vi "Get Interface Info.vi"(8 "error in (no error)":errorcluster, 10 "CASE":string, 11 "CSM-Helper in":refnum<class "CSM-Helper.lvclass">) -> (0 "error out":errorcluster, 1 "Response":T1[](array[typedef]), 2 "Array":T1[](array[typedef]), 3 "CSM-Helper out":refnum<class "CSM-Helper.lvclass">)   [LabVIEW 2017, in "CSM-Helper.lvclass"]
uses:
  CSM-Helper.lvclass
  Typedef/Def-Argument Info.ctl
  CSM-Helper.lvclass/CSM-Helper.ctl
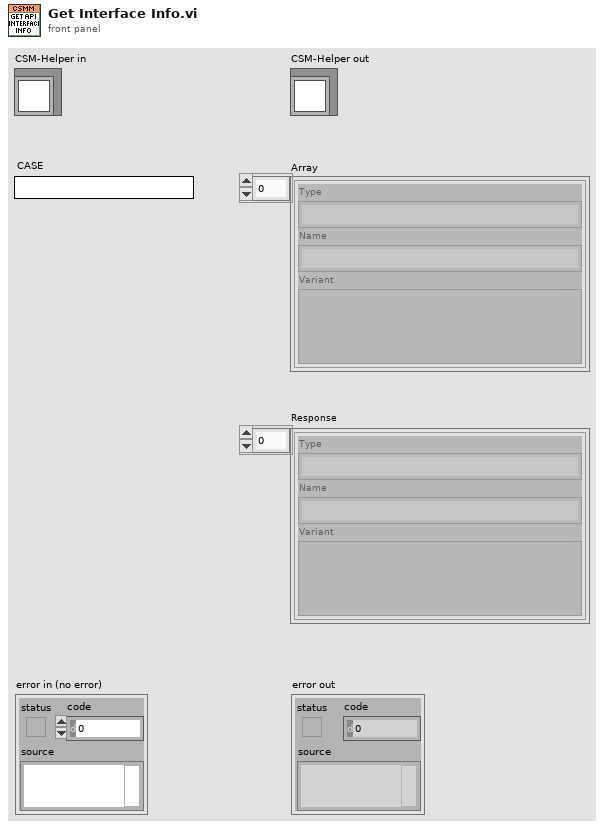
[diagram p1: front panel]
types:
  T1 = typedef "CSM-Helper.lvclass/Def-Argument Info.ctl" = cluster{"Type":string, "Name":string, "Variant":variant}
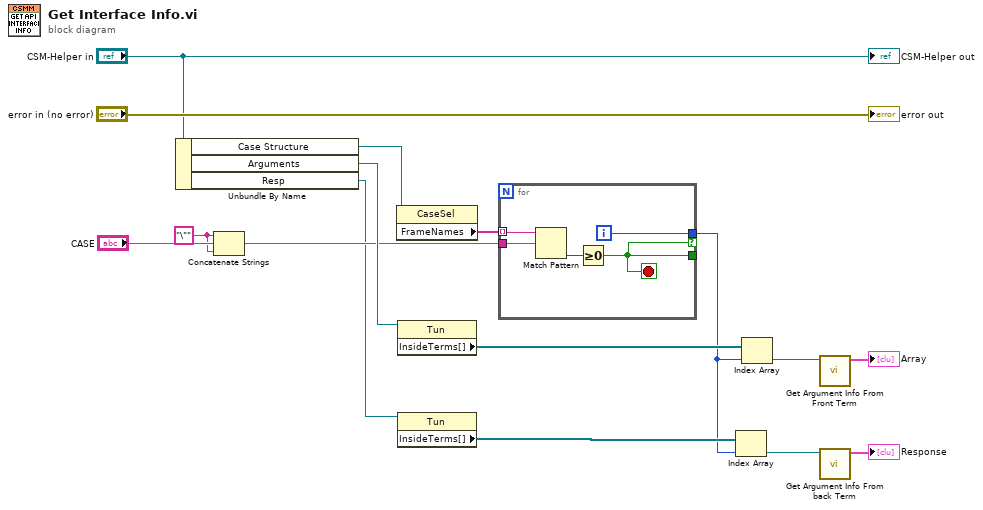
[diagram p0: block diagram]
diagram:
  w9 = "\"" ("string")
  n1 = Unbundle By Name("CSM-Helper in") -> ("Case Structure"=w14:refnum<vi>, "Arguments"=w13:refnum<vi>, "Resp"=w6:refnum<vi>)
  n2 = Concatenate Strings(w9, "CASE", w9) -> (w10:string)
  n3 = property class="CaseSel"(reference=w14) -> ("FrameNames"=w12:string[])  [unwired: 1 in, 2 out]
  n4 = property class="Tun"(reference=w13) -> ("InsideTerms[]"=w8:refnum<vi>[])  [unwired: 1 in, 2 out]
  n5 = property class="Tun"(reference=w6) -> ("InsideTerms[]"=w7:refnum<vi>[])  [unwired: 1 in, 2 out]
  n6 = for {
    tunnel: w12 -> [w21] mode=indexing
    tunnel: w10 -> [w20]
    tunnel: [w19] -> w5 if=w17
    tunnel: [w17] -> _
    i -> [w19]
    stop <- w17 stop-if-true
    n7 = Match Pattern(string=w21, regular expression=w20) -> (offset past match=w18:i32)  [unwired: 1 in, 3 out]
    n8 = Greater Or Equal To 0?(x=w18) -> (x >= 0?=w17:bool)
  }
  n9 = Index Array(array=w7, index=w5) -> (element=w2:refnum<vi>)
  n10 = Index Array(array=w8, index=w5) -> (element=w1:refnum<vi>)
  n11 = call "Get Argument Info From Front Term.vi"("Terminal in"=w1) -> ("Array"=→"Array":T1[])  [unwired: 10 in]
  n12 = call "Get Argument Info From back Term.vi"("Terminal in"=w2) -> ("Array"=→"Response":T1[])  [unwired: 10 in]
  "error out" <- "error in (no error)"
  "CSM-Helper out" <- "CSM-Helper in"
